vi "showrunningvis.vi"() -> ()   [LabVIEW 2019]
doc: "This example checks the execution state of all VIs in memory and displays the names and front panels of running VIs. You can configure it to display only top-level running VIs, only running subVIs, or both. A VI is in the \"Run top level\" state if its Run button was pressed and it hasn't finished executing. A VI is in the \"Running\" state if it is a subVI of a running VI. This VI uses application and VI property nodes to find the VIs in memory and read their execution state. \n \nUse this VI if you receive the \"Quitting will abort all running VIs\" when you try to exit LabVIEW and you have too many VIs to search manually to find out which one is running."
uses:
  <vilib>/addons/WireFlow/_WF_ProgressBar.llb/ProgressBar_WireFlow.lvclass
panel:
  in  "stop":bool
  out "VIs Found":string[][](table)
  in  "Find Sub-VIs":bool
  in  "Find Top-Level VIs":bool=TRUE
  in  "Show Front Panels":bool
  # "Select Help»Show Context Help and move the cursor over the VI icon to display help for this VI."
  # "This example checks the execution state of all VIs in memory and displays the names and front panels of \nrunning VIs. You can configure it to display only top-level running VIs, only running subVIs, or both. \nA VI is in the \"Run top level\" state if its Run button was pressed and it hasn't finished executing. A VI is \nin the \"Running\" state if it is a subVI of a running VI. This VI uses application and VI property nodes to find\nthe VIs in memory and read their execution state. \n \nUse this VI if you receive the \"Quitting will abort all running VIs\" when you try to exit LabVIEW \nand you have too many VIs to search manually to find out which one is running."
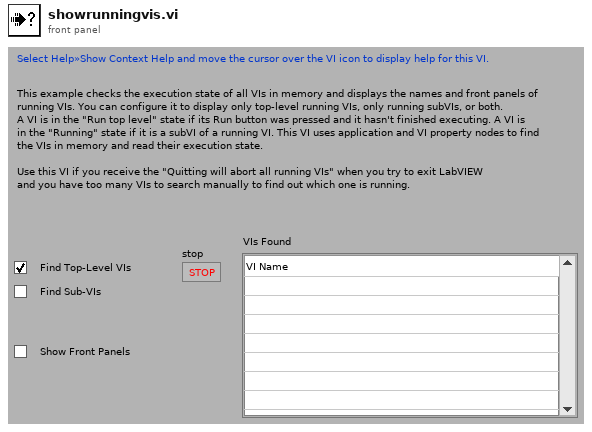
[diagram p1: front panel]
types:
  T1 = enum32{"Bad", "Idle", "Run top level", "Running"}
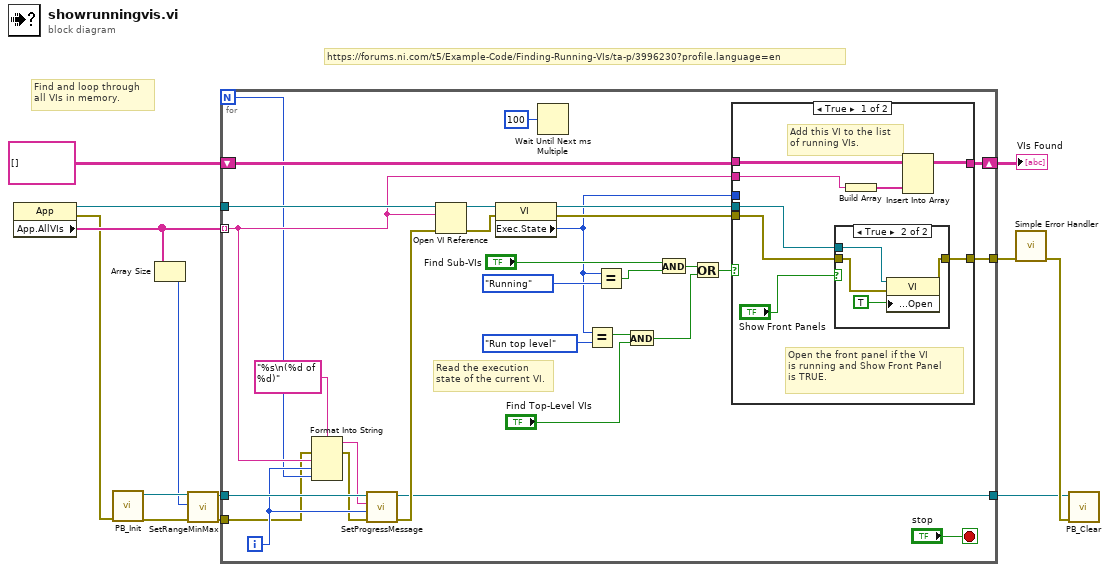
[diagram p0: block diagram]
diagram:
  # "https://forums.ni.com/t5/Example-Code/Finding-Running-VIs/ta-p/3996230?profile.language=en"
  # "Find and loop through\nall VIs in memory."
  n1 = property class="App"() -> (reference out=w13:refnum<vi>, error out=w4:errorcluster, "App.AllVIs"=w7:string[])  [unwired: 2 in]
  n2 = call <vilib>:"PB_Init.vi"("error in (no error)"=w4) -> ("error out"=w9:errorcluster, "WF-ProgressBar out"=w8:refnum<class "ProgressBar_WireFlow.lvclass">)  [unwired: 9 in]
  n3 = Array Size(array=w7) -> (size(s)=w6:i32)
  n4 = call-dynamic "SetRangeMinMax.vi"("error in (no error)"=w9, "Max (1)"=w6, "WF-ProgressBar in"=w8) -> ("error out"=w3:errorcluster, "WF-ProgressBar out"=w5:refnum<class "ProgressBar_WireFlow.lvclass">)  [unwired: 7 in]
  n5 = for {
    N -> [w18]
    tunnel: w7 -> [w19] mode=indexing
    tunnel: w13 -> [w42]
    shift-right: [w37] -> w10
    shift-left: string[][] [] ("Application:All VIs In Memory") -> [w38]
    tunnel: [w36] -> w11
    tunnel: w5 -> [w22]
    tunnel: w3 -> [w16]
    tunnel: [w23] -> w1
    i -> [w20]
    stop <- "stop" stop-if-true
    # "Read the execution\nstate of the current VI."
    n6 = Format Into String(format string="%s\n(%d of %d)", error in=w16, w19, w20, w18) -> (resulting string=w17:string, error out=w15:errorcluster)  [unwired: 1 in]
    n7 = call-dynamic "SetProgressMessage.vi"("error in (no error)"=w15, "Progress value (NaN no update)"=w20, "Message"=w17, "WF-ProgressBar in"=w22) -> ("error out"=w24:errorcluster, "WF-ProgressBar out"=w23:refnum<class "ProgressBar_WireFlow.lvclass">)  [unwired: 5 in, 1 out]
    n8 = Open VI Reference(application reference (local)=w42, vi path=w19, error in (no error)=w24) -> (vi reference=w43:refnum<vi>, error out=w41:errorcluster)  [unwired: 3 in]
    n9 = property class="VI"(reference=w43, error in=w41) -> (reference out=w39:refnum<vi>, error out=w40:errorcluster, "Exec.State"=w26:T1)
    n10 = Wait Until Next ms Multiple(millisecond multiple=u32 100) -> ()  [unwired: 1 out]
    n11 = Equal?(x=w26, y=T1."Run top level" ("Execution:State")) -> (x = y?=w31:bool)
    n12 = Equal?(x=w26, y=T1."Running" ("Execution:State")) -> (x = y?=w33:bool)
    n13 = And(x=w31, y="Find Top-Level VIs") -> (x .and. y?=w29:bool)
    n14 = And(x="Find Sub-VIs", y=w33) -> (x .and. y?=w28:bool)
    n15 = Or(x=w28, y=w29) -> (x .or. y?=w27:bool)
    n16 = case shown="True" w27 {
      tunnel: w40 -> [w51 w57]
      tunnel: w39 -> [w50 _]
      tunnel: w38 -> [w49 w58]
      tunnel: w19 -> [w45 _]
      tunnel: [w48 w58] -> w37
      tunnel: [w47 w57] -> w36
      tunnel: w26 -> [_ _]
      frame True {
        # "Add this VI to the list \nof running VIs."
        # "Open the front panel if the VI\nis running and Show Front Panel \nis TRUE."
        n17 = case shown="True" "Show Front Panels" {
          tunnel: w51 -> [w52 w55]
          tunnel: w50 -> [_ w54]
          tunnel: [w52 w53] -> w47
          frame False {
          }
          frame True {
            n18 = property class="VI"(reference=w54, error in=w55, "Front Panel.Open"=TRUE ("Front Panel Window:Open")) -> (error out=w53:errorcluster)  [unwired: 1 out]
          }
        }
        n19 = Build Array(w45) -> (w44:string[])
        n20 = Insert Into Array(array=w49, new element=w44) -> (w48:string[][])  [unwired: 2 in]
      }
      frame False {
      }
    }
  }
  "VIs Found" <- w10
  n21 = call <vilib>:"Simple Error Handler.vi"("error in (no error)"=w11) -> ("error out"=w2:errorcluster)  [unwired: 4 in, 4 out]
  n22 = call-dynamic "PB_Clear.vi"("error in (no error)"=w2, "WF-ProgressBar in"=w1) -> ()  [unwired: 8 in, 2 out]
